vi "Add Config File to Tree.vi"(8 "error in":errorcluster, 10 "HW Chassis List":refnum<class "Chassis BOM.lvclass">, 11 "FP Controls in":refnum<class "FP Controls.lvclass">) -> (0 "error out":errorcluster, 3 "FP Controls out":refnum<class "FP Controls.lvclass">)   [LabVIEW 2018, in "Configuration Grandmaster.lvlib" / "FP Controls.lvclass"]
uses:
  FP Controls.lvclass
  Class Chassis BOM/Chassis BOM.lvclass
  Class Chassis BOM/Chassis BOM.lvclass/Chassis BOM.ctl
  FP Controls.lvclass/FP Controls.ctl
  Class Chassis BOM/Read CfgFile.vi
  Class Chassis BOM/Read HW Mods.vi
  Class Chassis BOM/Read Chassis Alias.vi
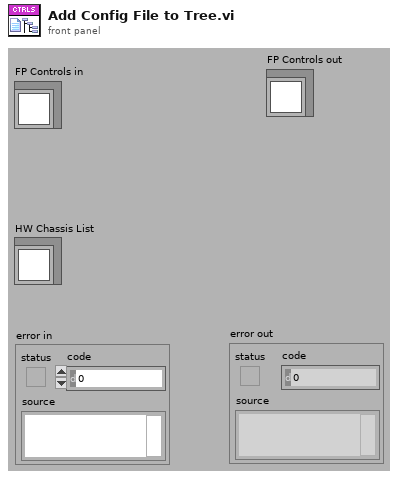
[diagram p1: front panel]
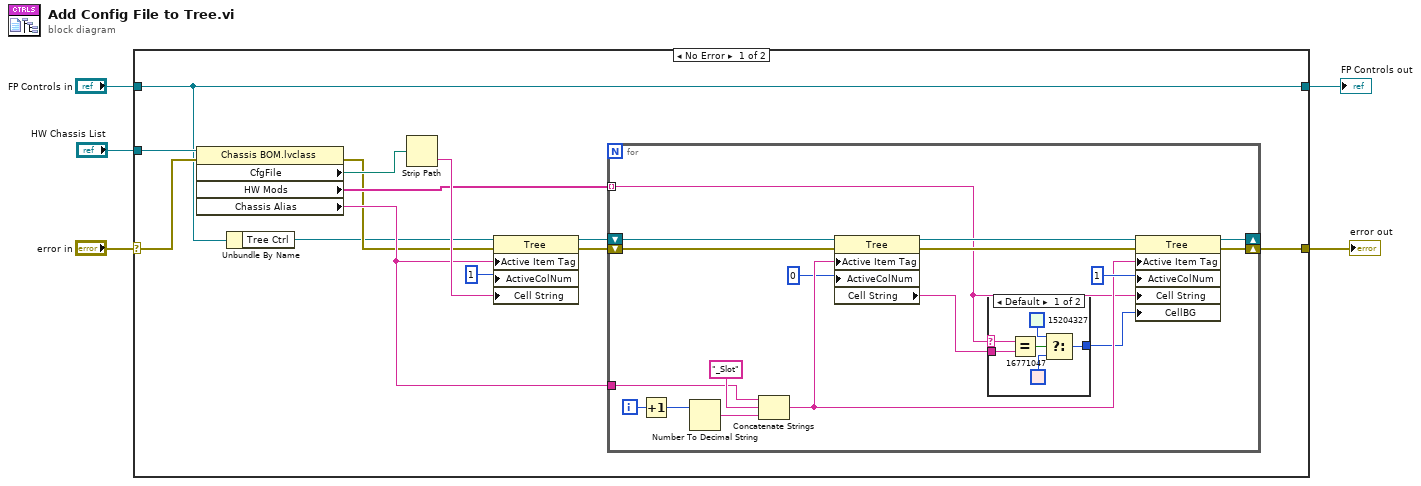
[diagram p0: block diagram]
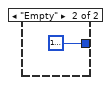
[diagram p2: hidden frame]
diagram:
  n1 = case shown="No Error" "error in" {
    selector: "error in" -> [w7 w44]
    tunnel: "HW Chassis List" -> [w14 _]
    tunnel: [w8 w44] -> w4
    tunnel: "FP Controls in" -> [w6 w43]
    tunnel: [w6 w43] -> w1
    frame No Error {
      n2 = property class="Chassis BOM.lvclass"(reference=w14, error in=w7) -> (error out=w10:errorcluster, "CfgFile"=w13:path, "HW Mods"=w12:string[], "Chassis Alias"=w11:string)  [unwired: 1 out]
      n3 = Unbundle By Name(w6) -> ("Tree Ctrl"=w9:refnum<vi>)
      n4 = Strip Path(path=w13) -> (name=w15:string)  [unwired: 1 out]
      n5 = property class="Tree"(reference=w9, error in=w10, "Active Item Tag"=w11, "ActiveColNum"=1 ("Active Cell:Active Column Number"), "Cell String"=w15) -> (reference out=w16:refnum<vi>, error out=w17:errorcluster)
      n6 = for {
        shift-right: [w34] -> w8
        shift-left: w17 -> [w24]
        shift-right: [w35] -> _
        shift-left: w16 -> [w27]
        tunnel: w11 -> [w30]
        tunnel: w12 -> [w19] mode=indexing
        i -> [w28]
        n7 = Increment(x=w28) -> (x+1=w29:i32)
        n8 = Number To Decimal String(number=w29) -> (decimal integer string=w33:string)  [unwired: 1 in]
        n9 = Concatenate Strings(w30, "_Slot" ("string"), w33) -> (w23:string)
        n10 = property class="Tree"(reference=w27, error in=w24, "Active Item Tag"=w23, "ActiveColNum"=0 ("Active Cell:Active Column Number")) -> (reference out=w26:refnum<vi>, error out=w25:errorcluster, "Cell String"=w21:string)
        n11 = case shown="Default" w19 {
          selector: w19 -> [w36 _]
          tunnel: w21 -> [w41 _]
          tunnel: [w37 u32 16777225] -> w20
          frame Default {
            n12 = Equal?(x=w36, y=w41) -> (x = y?=w40:bool)
            n13 = Select(t=u32 15204327, s=w40, f=u32 16771047) -> (s? t:f=w37:u32)
          }
          frame "Empty" {
          }
        }
        n14 = property class="Tree"(reference=w26, error in=w25, "Active Item Tag"=w23, "ActiveColNum"=1 ("Active Cell:Active Column Number"), "Cell String"=w19, "CellBG"=w20) -> (reference out=w35:refnum<vi>, error out=w34:errorcluster)
      }
    }
    frame Error {
    }
  }
  "error out" <- w4
  "FP Controls out" <- w1
